vi "Netburner_cntl3.vi"() -> ()   [LabVIEW 2013]
panel:
  out "#  Bytes Read last":u32
  out "ADC last":string
  in  "Number of Cycles":i32=100
  out "ADC result":string
  out "#  Bytes Read":u32
  in  "DAC, ADC String":string="0 1. 1 -1. 0 100"
  out "Error Out":errorcluster={"status"=FALSE, "code"=1073676294, "source"="VISA Read in Netburner_RD.vi->Netburner_cntl.vi"}
  in  "Error In (none)":errorcluster
  in  "COM Port #":refnum<visa-resource-name>="COM3"
  # "Netburner ADC/DAC Test Interface"
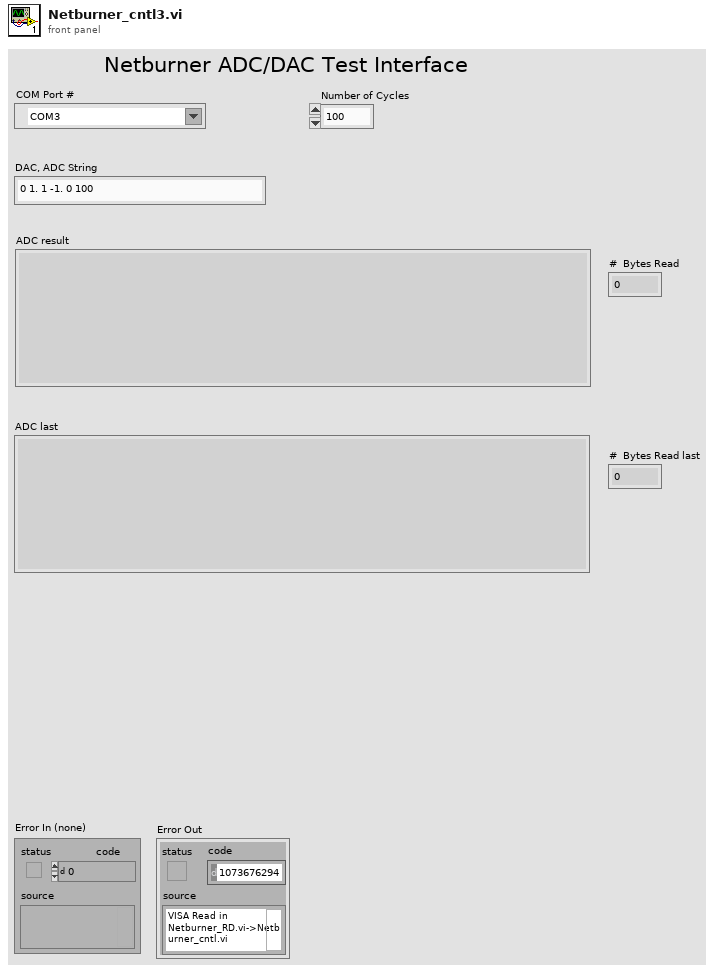
[diagram p1: front panel]
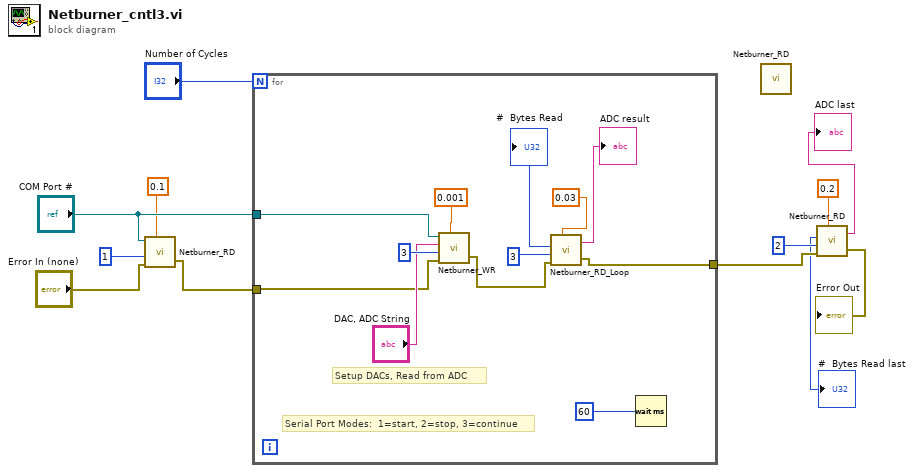
[diagram p0: block diagram]
diagram:
  n1 = call "Netburner_RD.vi"("VISA resource name (COM Port #)"="COM Port #", "Mode (0)"=1, "Error In (no error)"="Error In (none)", "Wait (sec)"=0.1) -> ("Error Out"=w10:errorcluster)  [unwired: 2 out]
  n2 = for {
    N: "Number of Cycles" -> [_]
    tunnel: "COM Port #" -> [w21]
    tunnel: w10 -> [w19]
    tunnel: [w18] -> w6
    # "Serial Port Modes:  1=start, 2=stop, 3=continue"
    # "Setup DACs, Read from ADC"
    n3 = call "Netburner_WR.vi"("VISA resource name (COM Port #)"=w21, "String to Send"="DAC, ADC String", "Mode (0)"=3, "Error In (no error)"=w19, "Wait (sec)"=0.001) -> ("Error Out"=w17:errorcluster)  [unwired: 1 in]
    n4 = call "Netburner_RD_Loop.vi"("Mode (0)"=3, "Error In (no error)"=w17, "Wait (sec)"=0.03) -> ("#  Bytes Read"=→"#  Bytes Read":u32, "Return String from Device"=→"ADC result":string, "Error Out"=w18:errorcluster)  [unwired: 1 in]
    n5 = Wait (ms)(milliseconds to wait=60) -> ()  [unwired: 1 out]
  }
  n6 = call "Netburner_RD.vi"() -> ()  [unwired: 4 in, 3 out]
  n7 = call "Netburner_RD.vi"("Mode (0)"=2, "Error In (no error)"=w6, "Wait (sec)"=0.2) -> ("Number of Bytes Received"=→"#  Bytes Read last":u32, "Return String from Device"=→"ADC last":string, "Error Out"=→"Error Out":errorcluster)  [unwired: 1 in]
